vi "Pre Launch Init.vi"(11 "Settings in":refnum<class "Settings.lvclass">) -> (0 "error out":errorcluster, 3 "Settings out":refnum<class "Settings.lvclass">)   [LabVIEW 2015, in "Item Actor.lvlib" / "Settings.lvclass"]
doc: "(<B>Filename</B>: Actor Framework.lvlib:Actor.lvclass:Pre Launch Init.vi)\n\nDefines behavior that occurs after the Launch Nested Actor method is invoked but before the actor's Actor Core method begins running.\n\nBy default, this method does nothing. A descendant class may override it to define behavior."
uses:
  Settings.lvclass
  Settings.lvclass/Settings.ctl
  VI Store/VIStore Actor/VIStore.lvclass
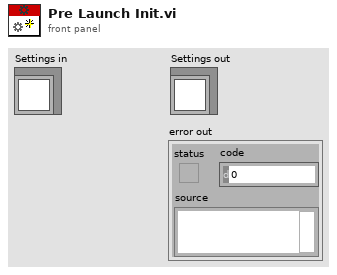
[diagram p1: front panel]
types:
  T1 = typedef "Item Actor.lvlib/Settings.lvclass/Settings Data.ctl" = cluster{"Categories Path":path, "Resizable":bool}
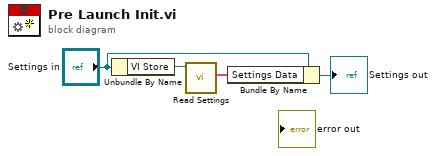
[diagram p0: block diagram]
diagram:
  n1 = Unbundle By Name("Settings in") -> ("VI Store"=w4:refnum<class "VIStore.lvclass">)
  n2 = call "Read Settings.vi"("VIStore in"=w4) -> ("Settings Data"=w1:T1)  [unwired: 8 in, 2 out]
  n3 = Bundle By Name(cluster="Settings in", "Settings Data"=w1) -> (→"Settings out":refnum<class "Settings.lvclass">)
